vi "Write AI channel.vi"(8 "error in":errorcluster, 10 "AI channel":refnum<class "AI Channel.lvclass">, 11 "analog input mode in":refnum<class "Analog Input Mode.lvclass">) -> (0 "error out":errorcluster, 3 "analog input mode out":refnum<class "Analog Input Mode.lvclass">)   [LabVIEW 2017, in "Scan Engine Scripting.lvlib" / "Analog Input Mode.lvclass"]
doc: "Writes the analog input channel class that is stored in the private data of the analog input mode."
uses:
  Analog Input Vrms Mode/Analog Input Mode.lvclass
  Channel Classes/AI Channel/AI Channel.lvclass
  Analog Input Vrms Mode/Analog Input Mode.lvclass/Analog Input Mode.ctl
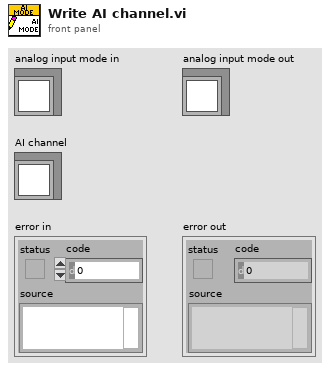
[diagram p1: front panel]
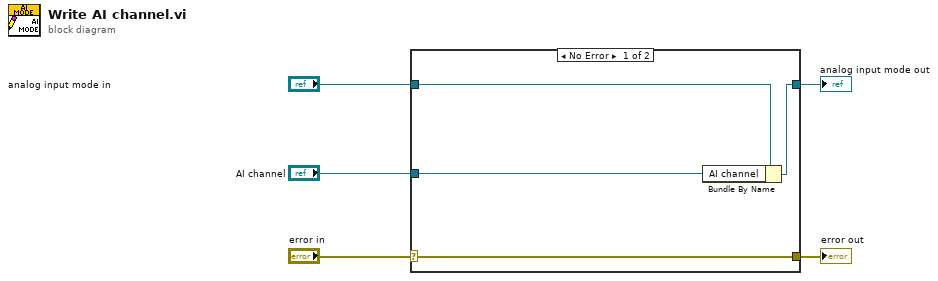
[diagram p0: block diagram]
diagram:
  n1 = case shown="No Error" "error in" {
    selector: "error in" -> [w9 w10]
    tunnel: [w9 w10] -> w4
    tunnel: [w7 w11] -> w2
    tunnel: "analog input mode in" -> [w8 w11]
    tunnel: "AI channel" -> [w6 _]
    frame No Error {
      n2 = Bundle By Name(cluster=w8, "AI channel"=w6) -> (w7:refnum<class "Analog Input Mode.lvclass">)
    }
    frame Error {
    }
  }
  "error out" <- w4
  "analog input mode out" <- w2
